vi "OpenNetworkStreamReader.vi"(6 "E-Stop DVR":refnum<data-value>, 8 "error in (no error)":errorcluster, 11 "Reader Parameters":T1={"reader name"="", "writer url"="", "reader buffer size"=-1}) -> (0 "error out":errorcluster, 2 "Time Opened":timestamp, 3 "Reader Endpoint":refnum<k21>, 4 "Aborted?":bool)   [LabVIEW 2013, in "NetworkStreamReader.lvclass"]
doc: "Opens a network stream reader endpoint. This VI persistently tries to open the connection until it is successful or the e-stop is triggered by-reference (data value reference). The e-stop will be triggered by the Close method of the owning Object.\n\nJared Kirschner, 2012."
uses:
  NetworkStreamReader.lvclass
  ReaderParameters.ctl
  Shared/ElapsedTimeMessage.ctl
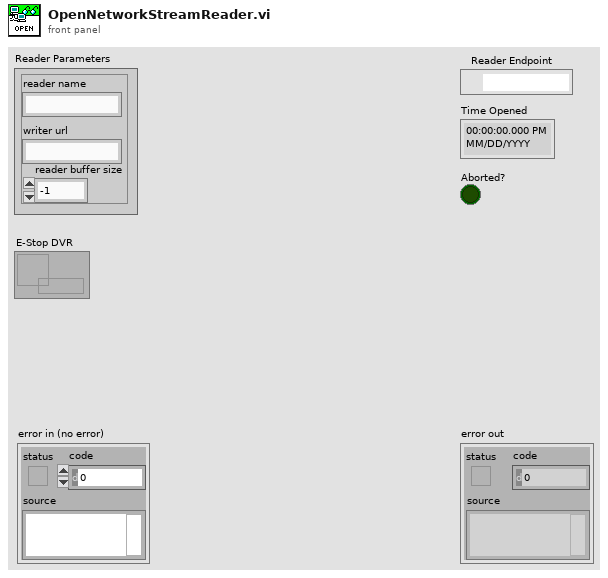
[diagram p1: front panel]
types:
  T1 = typedef "NetworkStreamReader.lvclass/ReaderParameters.ctl" = cluster{"reader name":string, "writer url":string, "reader buffer size":i32}
  T2 = typedef "ElapsedTimeMessage.ctl" = cluster{"Data":variant, "Elapsed Time (s)":dbl}
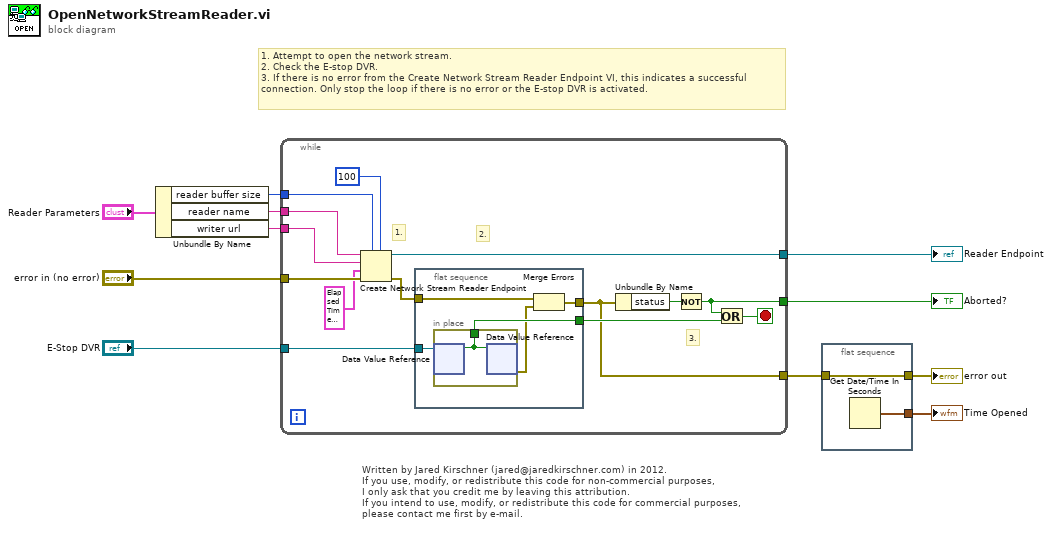
[diagram p0: block diagram]
diagram:
  # "1. Attempt to open the network stream.\n2. Check the E-stop DVR.\n3. If there is no error from the Create Network Stream Reader Endpoint VI, this indicates a successful\nconnection. Only stop the loop if there is no error or the E-stop DVR is activated."
  # "Written by Jared Kirschner (jared@jaredkirschner.com) in 2012.\nIf you use, modify, or redistribute this code for non-commercial purposes,\nI only ask that you credit me by leaving this attribution.\nIf you intend to use, modify, or redistribute this code for commercial purposes,\nplease contact me first by e-mail."
  n1 = Unbundle By Name("Reader Parameters") -> ("reader buffer size"=w9:i32, "reader name"=w8:string, "writer url"=w7:string)
  n2 = while {
    tunnel: "error in (no error)" -> [w25]
    tunnel: [w23] -> w1
    tunnel: w9 -> [w22]
    tunnel: w8 -> [w20]
    tunnel: w7 -> [w19]
    tunnel: "E-Stop DVR" -> [w15]
    tunnel: [w17] -> w5
    tunnel: [w12] -> w3
    stop <- w18 stop-if-true
    # "3."
    # "2."
    # "1."
    n3 = Create Network Stream Reader Endpoint(5:100 ("timeout in ms (-1)"), 7:w22, 8:w25, 9:T2 {"Data"=variant, "Elapsed Time (s)"=0.0} ("variant"), 10:w19, 11:w20) -> (0:w16:errorcluster, 3:w23:refnum<k21>)  [unwired: 1 in]
    n4 = flat-sequence {
      tunnel: [w30] -> w13
      tunnel: [w29] -> w12
      tunnel: w16 -> [w27]
      tunnel: w15 -> [w26]
      frame #0 {
        n5 = in-place {
          in-place-border: [w31] -> w30
          n6 = in-place-dvr #1(w26) -> (w31:bool)  [unwired: 1 out]
          n7 = in-place-dvr #1(w31) -> (w28:errorcluster)  [unwired: 1 out]
        }
        n8 = Merge Errors(w27, w28) -> (w29:errorcluster)
      }
    }
    n9 = Unbundle By Name(w12) -> ("status"=w14:bool)
    n10 = Not(x=w14) -> (.not. x?=w17:bool)
    n11 = Or(x=w17, y=w13) -> (x .or. y?=w18:bool)
  }
  "Aborted?" <- w5
  "Reader Endpoint" <- w1
  n12 = flat-sequence {
    tunnel: w3 -> [w33]
    tunnel: [w33] -> w2
    tunnel: [w32] -> w4
    frame #0 {
      n13 = Get Date/Time In Seconds() -> (seconds since 1Jan1904=w32:timestamp)
    }
  }
  "error out" <- w2
  "Time Opened" <- w4
